vi "Set Host IP Address.vi"(10 "Host IP Address":string, 11 "Reply Protocol DataSocket in":refnum<class "Reply Protocol DataSocket.lvclass">) -> (3 "Reply Protocol DataSocket out":refnum<class "Reply Protocol DataSocket.lvclass">)   [LabVIEW 2023, in "HAL GOOP4.lvlib" / "Reply Protocol DataSocket.lvclass"]
uses:
  Reply Protocol DataSocket.lvclass
  Reply Protocol DataSocket.lvclass/Reply Protocol DataSocket.ctl
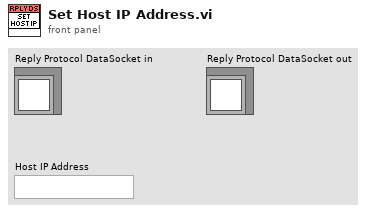
[diagram p1: front panel]
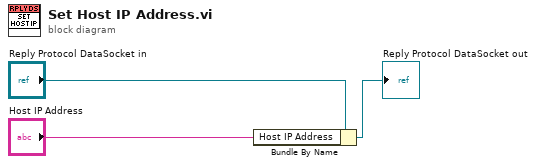
[diagram p0: block diagram]
diagram:
  n1 = Bundle By Name(cluster="Reply Protocol DataSocket in", "Host IP Address"="Host IP Address") -> (→"Reply Protocol DataSocket out":refnum<class "Reply Protocol DataSocket.lvclass">)
